vi "SwisssSPAD Live_Histogram Dynanic Event.vi"(8 "error in":errorcluster) -> (0 "error out":errorcluster, 2 "User Event out":refnum<user-event>)   [LabVIEW 2021]
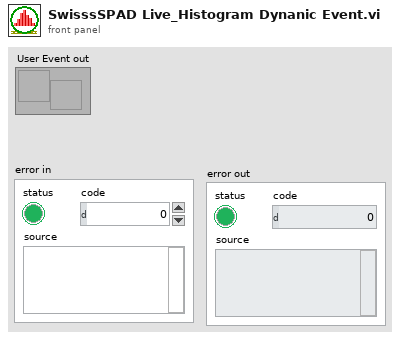
[diagram p1: front panel]
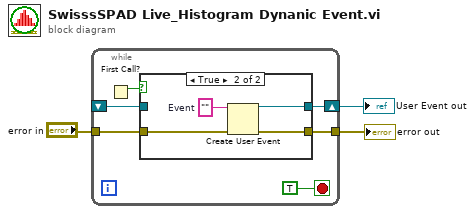
[diagram p0: block diagram]
diagram:
  n1 = while {
    shift-right: [w9] -> w3
    shift-left: _ -> [w6]
    tunnel: [w5] -> w2
    tunnel: "error in" -> [w4]
    stop <- TRUE stop-if-true
    n2 = First Call?() -> (First Call?: T/F=w7:bool)
    n3 = case shown="True" w7 {
      tunnel: [w11 w15] -> w9
      tunnel: w6 -> [w11 _]
      tunnel: [w10 w13] -> w5
      tunnel: w4 -> [w10 w12]
      frame False {
      }
      frame True {
        w14 = ""  # Event
        n4 = Create User Event(user event datatype=w14, error in=w12) -> (user event=w15:refnum<user-event>, error out=w13:errorcluster)
      }
    }
  }
  "error out" <- w2
  "User Event out" <- w3
